vi "Execute.vi"(8 "error in":errorcluster, 10 "Command in":refnum<class "Command.lvclass">, 11 "Object In":refnum<class>) -> (0 "error out":errorcluster, 3 "Object Out":refnum<class>)   [LabVIEW 2014, in "Command.lvclass"]
doc: "This is the concrete method for executing commands."
uses:
  Command.lvclass
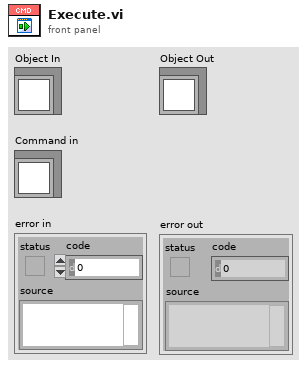
[diagram p1: front panel]
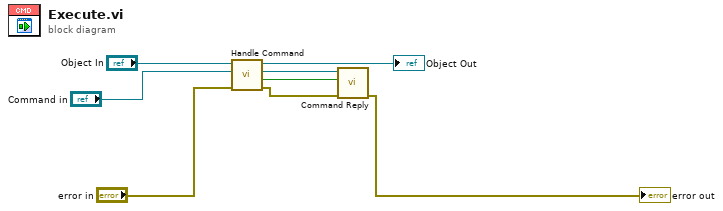
[diagram p0: block diagram]
diagram:
  n1 = call-dynamic "Handle Command.vi"("error in (no error)"="error in", "CMD in"="Command in", "Object In"="Object In") -> ("error out"=w3:errorcluster, "Command Successful?"=w8:bool, "CMD out"=w5:refnum<class "Command.lvclass">, "Object Out"=→"Object Out":refnum<class>)  [unwired: 5 in]
  n2 = call "Command Reply.vi"("error in"=w3, "cmd successful"=w8, "CMD in"=w5) -> ("error out"=→"error out":errorcluster)  [unwired: 7 in, 1 out]
